vi "MDOAcquire Data from х502.vi"(8 "error in (no error)":errorcluster, 10 "Coeff":T2={"Coeff_U"=300.0, "Offset_U"=0.0, "Coeff_I"=23.5, "Offset_I"=0.15}, 11 "Hardware Configuration":T1 {"SyncMode" items=["INTERNAL"=0, "EXTERNAL_MASTER"=1, "DI_SYN1_RISE"=2, "DI_SYN1_FALL"=3, "DI_SYN2_RISE"=6, "DI_SYN2_FALL"=7]}) -> (0 "error out":errorcluster, 2 "Ток":dbl[](graph), 3 "Напряжение":dbl[](graph))   [LabVIEW 2012]
uses:
  controls/Coeff.ctl
  controls/MDOHW Configuration.ctl
  <vilib>/Analysis/3filter.llb/Filter Passband Type.ctl
  <vilib>/Analysis/3filter.llb/Butterworth Filter (DBL).vi
  <vilib>/Analysis/NI_AALBase.lvlib
panel:
  out "Gauge":dbl(knob) scale=0.0..10.0
  in  "stop":bool
  out "din_data_size":u32
  out "DIN":u32[](array[numeric]) format="%b"
  in  "IP Addr":string="192.168.0.1"
  out "MCU ver":string
  in  "Отображать за время":dbl=100.0 min=10.0 step=1.0
  out "Установленная частота синхронного ввода DIN":dbl=2.0 min=2.0 max=2000000.0 format="%#_8f"
  in  "Частота синхронного ввода DIN":dbl=20000.0 min=1.0 max=2000000.0 format="%#_8f"
  out "FPGA Ver":string
  out "Установленная частота на канал":dbl=2.0 min=2.0 max=2000000.0 format="%#_8f"
  out "Установленная частота сбора":dbl=2.0 min=2.0 max=2000000.0 format="%#_8f"
  in  "Частота сбора на канал":dbl=50000.0 min=2.0 max=2000000.0 format="%#_8f"
  in  "Частота сбора (Гц)":dbl=100000.0 min=2.0 max=2000000.0 format="%#_8f"
  out "PldaVer":u8
  out "Serial":string
  out "Name":string
  # "Ожидание триггера"
  # "Информация о плате"
  # "Настройки модуля"
  # "Устанавливаемое"
  # "Установленное"
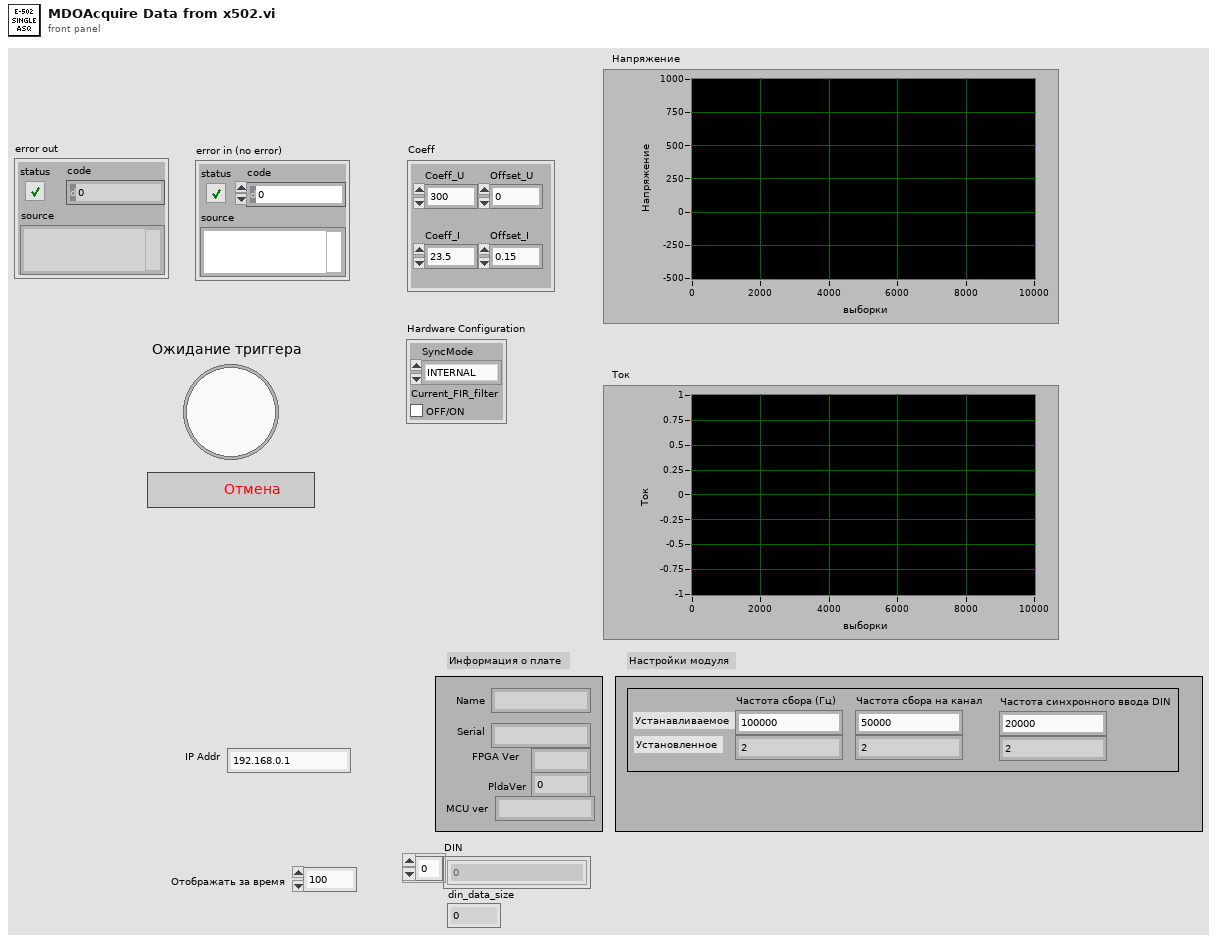
[diagram p1: front panel]
types:
  T1 = typedef "MDOHW Configuration.ctl" = cluster{"SyncMode":u32, "Current_FIR_filter":bool}
  T2 = typedef "Coeff.ctl" = cluster{"Coeff_U":dbl, "Offset_U":dbl, "Coeff_I":dbl, "Offset_I":dbl}
  T3 = cluster{"PhyCh":u32, "Avg":u32, "Mode":u32, "Range":u32}[]
  T4 = typedef "NI_AALBase.lvlib/Filter Passband Type.ctl" = enum32{"Lowpass", "Highpass", "Bandpass", "Bandstop"}
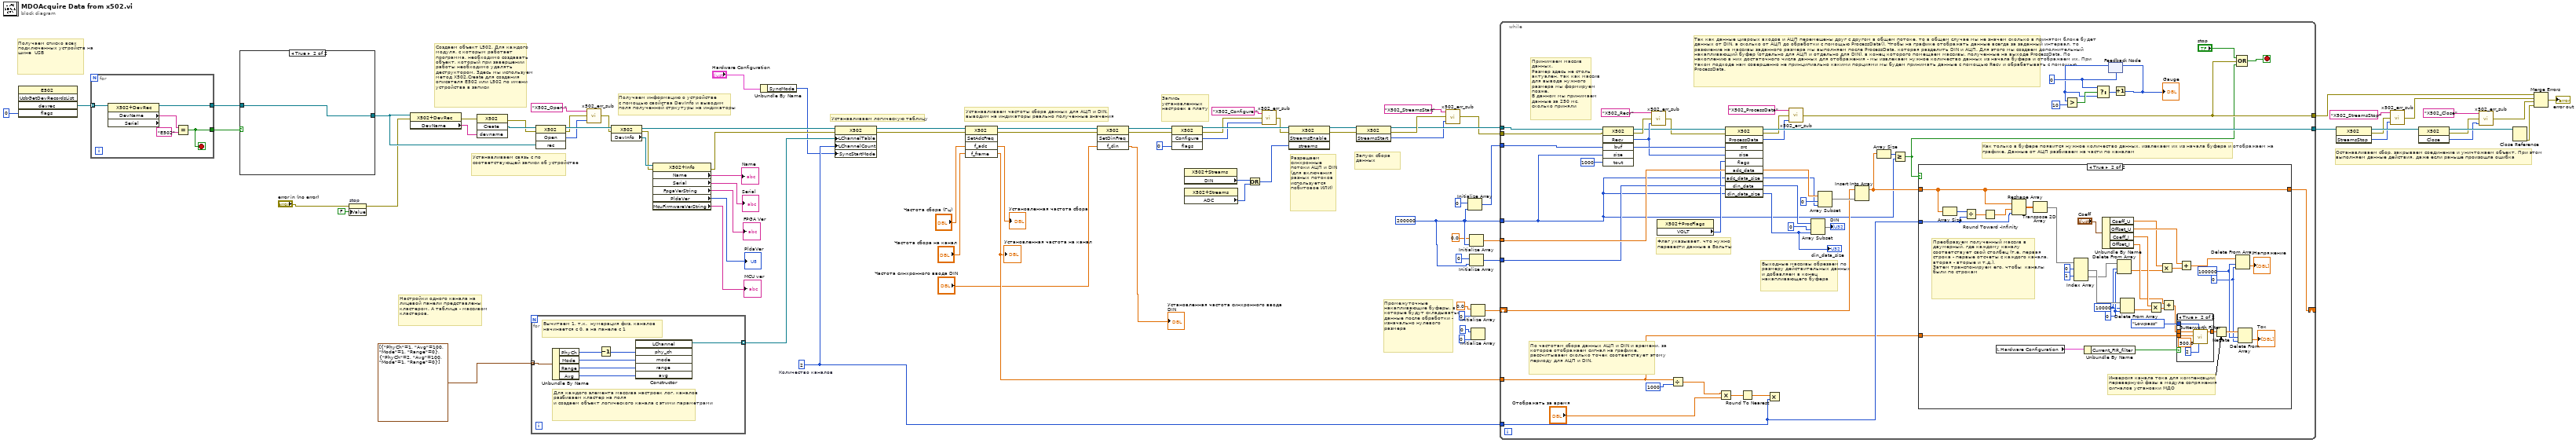
[diagram p0: block diagram]
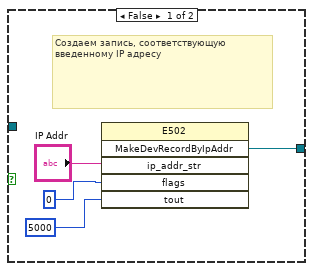
[diagram p4: hidden frame]
diagram:
  w85 = u32 2  # Количество каналов
  w81 = u32 200000 ("element")
  # "Промежуточные накапливающие буферы, в которые будут складываться данные после обработки - изначально нулевого размера"
  # "Получаем списко всех подключенных устройств на шине  USB"
  # "Останавливаем сбор, закрываем соединение и уничтожаем объект. При этом выполняем данные действия, даже если раньше произошла ошибка"
  # "Запуск сбора данных"
  # "Разрешаем синхронные потоки АЦП и DIN (для включения разных потоков используется побитовое ИЛИ)"
  # "Запись установленных настроек в плату"
  # "Устанавливаем частоты сбора данных для АЦП и DIN,\nвыводим на индикаторы реально полученные значения"
  # "Устанавливаем логическую таблицу"
  # "Настройки одного канала на лицевой панели представлены кластером. А таблица - массивом кластеров."
  # "Создаем объект L502. Для каждого модуля, с которым работает программа, необходимо создавать объект, который при завершении работы необходимо удалять деструктором. Здесь мы используем метод X502.Create для создания описателя E502 или L502 по имени устройства в записи"
  # "Получаем информацию о устройстве \nс помощью свойства DevInfo и выводим\nполя полученной стркутуры на индикаторы"
  # "Устанавливаем связь с по соответствующей записи об устройстве"
  n1 = invoke class="E502" method="UsbGetDevRecordsList"("flags"=0) -> ("devrec"=w15:refnum<k24>[])  [unwired: 4 in, 4 out]
  n2 = for {
    tunnel: w15 -> [w90] mode=indexing
    tunnel: [w89] -> w13
    tunnel: [w86] -> w14
    stop <- w86 stop-if-true
    n3 = property class="X502+DevRec" props=["DevName", "Serial"](reference=w90) -> (reference out=w89:refnum<k24>, "DevName"=w88:string)  [unwired: 1 in, 2 out]
    n4 = Equal?(x=w88, y="E502") -> (x = y?=w86:bool)
  }
  n5 = case shown="True" w14 {
    tunnel: [w91 w95] -> w22
    tunnel: w13 -> [_ w95]
    frame False {
      # "Создаем запись, соответствующую введенному IP адресу"
      n6 = invoke class="E502" method="MakeDevRecordByIpAddr"("ip_addr_str"="IP Addr", "flags"=0, "tout"=5000) -> ("MakeDevRecordByIpAddr"=w91:refnum<k24>)  [unwired: 3 in, 5 out]
    }
    frame True {
    }
  }
  n7 = property on="stop" class="Bool (strict)"(error in="error in (no error)", "Value"=FALSE ("Visible")) -> (error out=w10:errorcluster)  [unwired: 1 in, 1 out]
  n8 = property class="X502+DevRec"(reference=w22, error in=w10) -> (error out=w17:errorcluster, "DevName"=w53:string)  [unwired: 1 out]
  n9 = invoke class="X502" method="Create"(error in=w17, "devname"=w53) -> (error out=w52:errorcluster, "Create"=w54:refnum<k24>)  [unwired: 2 in, 2 out]
  n10 = for {
    tunnel: T3 [{"PhyCh"=1, "Avg"=100, "Mode"=1, "Range"=0}, {"PhyCh"=2, "Avg"=100, "Mode"=1, "Range"=0}] ("Логические каналы") -> [w102] mode=indexing
    tunnel: [w96] -> w77 mode=indexing
    # "Вычитаем 1, т.к.  нумерация физ. каналов начинается с 0, а на панеле с 1"
    # "Для каждого элемента массива настроек лог. каналов разбиваем кластер на поля\nи создаем объект логического канала с этими параметрами"
    n11 = Unbundle By Name(w102) -> ("PhyCh"=w101:u32, "Mode"=w99:u32, "Range"=w98:u32, "Avg"=w97:u32)
    n12 = Decrement(x=w101) -> (x-1=w100:u32)
    n13 = constructor class="X502+LChannel"("phy_ch"=w100, "mode"=w99, "range"=w98, "avg"=w97) -> (reference out=w96:refnum<k24>)  [unwired: 3 in, 6 out]
  }
  n14 = invoke class="X502" method="Open"(reference=w54, error in=w52, "rec"=w22) -> (reference out=w57:refnum<k24>, error out=w50:errorcluster, "Open"=w51:i32)  [unwired: 1 in, 1 out]
  n15 = call "x502_err_sub.vi"("Error code"=w51, "error in (no error)"=w50, "Error descr"="X502_Open ") -> ("error out"=w48:errorcluster)
  n16 = property class="X502"(reference=w57, error in=w48) -> (reference out=w58:refnum<k24>, error out=w46:errorcluster, "DevInfo"=w47:refnum<k24>)
  n17 = property class="X502+Info"(reference=w47, error in=w46) -> (error out=w23:errorcluster, "Name"=→"Name":string, "Serial"=→"Serial":string, "FpgaVerString"=→"FPGA Ver":string, "PldaVer"=→"PldaVer":u8, "McuFirmwareVerString"=→"MCU ver":string)  [unwired: 1 out]
  n18 = Unbundle By Name("Hardware Configuration") -> ("SyncMode"=w1:u32)
  n19 = property class="X502"(reference=w58, error in=w23, "LChannelTable"=w77, "LChannelCount"=w85, "SyncStartMode"=w1) -> (reference out=w59:refnum<k24>, error out=w60:errorcluster)
  n20 = invoke class="X502" method="SetAdcFreq"(reference=w59, error in=w60, "f_adc"="Частота сбора (Гц)", "f_frame"="Частота сбора на канал") -> (reference out=w64:refnum<k24>, error out=w65:errorcluster, "f_adc"=→"Установленная частота сбора":dbl, "f_frame"=w78:dbl)  [unwired: 1 in, 1 out]
  "Установленная частота на канал" <- w78
  n21 = invoke class="X502" method="SetDinFreq"(reference=w64, error in=w65, "f_din"="Частота синхронного ввода DIN") -> (reference out=w69:refnum<k24>, error out=w70:errorcluster, "f_din"=→"Установленная частота синхронного ввода DIN":dbl)  [unwired: 1 in, 1 out]
  n22 = invoke class="X502" method="Configure"(reference=w69, error in=w70, "flags"=0) -> (reference out=w71:refnum<k24>, error out=w40:errorcluster, "Configure"=w38:i32)  [unwired: 1 in, 1 out]
  n23 = property class="X502+Streams"() -> ("DIN"=w32:u32)  [unwired: 2 in, 2 out]
  n24 = property class="X502+Streams"() -> ("ADC"=w68:u32)  [unwired: 2 in, 2 out]
  n25 = Or(x=w32, y=w68) -> (x .or. y?=w31:u32)
  n26 = call "x502_err_sub.vi"("Error code"=w38, "error in (no error)"=w40, "Error descr"="X502_Configure ") -> ("error out"=w39:errorcluster)
  n27 = invoke class="X502" method="StreamsEnable"(reference=w71, error in=w39, "streams"=w31) -> (reference out=w72:refnum<k24>, error out=w73:errorcluster)  [unwired: 1 in, 2 out]
  n28 = invoke class="X502" method="StreamsStart"(reference=w72, error in=w73) -> (reference out=w34:refnum<k24>, error out=w36:errorcluster, "StreamsStart"=w8:i32)  [unwired: 1 in]
  n29 = call "x502_err_sub.vi"("Error code"=w8, "error in (no error)"=w36, "Error descr"="X502_StreamsStart") -> ("error out"=w33:errorcluster)
  n30 = Initialize Array(u32 0 ("element"), w81) -> (w82:u32[])
  n31 = Initialize Array(0.0 ("element"), w81) -> (w84:dbl[])
  n32 = Initialize Array(u32 0 ("element"), w81) -> (w83:u32[])
  n33 = Initialize Array(0.0 ("element"), u32 0 ("element")) -> (w3:dbl[])
  n34 = Initialize Array(u32 0 ("element"), u32 0 ("element")) -> ()  [unwired: 1 out]
  n35 = while {
    tunnel: w85 -> [w149]
    tunnel: w84 -> [w148]
    tunnel: w83 -> [w147]
    tunnel: w82 -> [w146]
    tunnel: w81 -> [w104]
    tunnel: w78 -> [w113]
    tunnel: w34 -> [w145]
    tunnel: w33 -> [w144]
    tunnel: [w143] -> w30
    tunnel: [w121] -> w18
    shift-right: [w107] -> _
    shift-left: w3 -> [w108]
    stop <- w120 stop-if-true
    w116 = 0
    # "Так как данные цивроых входов и АЦП перемешены друг с другом в общем потоке, то в общем случае мы не значем сколько в принятом блоке будет данных от DIN, а сколько от АЦП до обработки с помощью ProcessData(). Чтобы на графике отображать данные всегда за заданный интервал, то разюиение на массивы заданного размера мы выполняем после ProcessData, которая разделить DIN и АЦП. Для этого мы создаем дополнительный накапливающий буфер (отдельно для АЦП и отдельно для DIN), в конец которого помещаем массивы, полученные на выходе ProcessData. По накоплению в них достаточного числа данных для отображения - мы извлекаем нужное количество данных из начала буфера и отображаем их. При таком подходе нам совершенно не принципиально какими порциями мы будем принимать данные с помощью Recv и обрабатывать с помощью ProcessData."
    # "Как только в буфере появится нужное количество данных, извлекаем их из начала буфера и отображаем на графике. Данные от АЦП разбиваем на части по каналам"
    # "По частотам сбора данных АЦП и DIN и времени, за которое отображаем сигнал на графике, рассчитываем сколько точек соответствует этому периоду для АЦП и DIN."
    # "Выходные массивы обрезаем по размеру действительных данных и добавляем в конец накапливающего буфера"
    # "Флаг указывает, что нужно перевести данные в Вольты"
    # "Принимаем массив данных.\nРазмер здесь не столь актуален, так как массив для вывода нужного размера мы формируем позже.\nВ данном мы принимаем данные за 250 мс, сколько приняли"
    n36 = invoke class="X502" method="Recv"(reference=w145, error in=w144, "buf"=w146, "size"=w104, "tout"=u32 1000 ("element")) -> (reference out=w124:refnum<k24>, error out=w130:errorcluster, "Recv"=w129:i32, "buf"=w142:u32[])  [unwired: 1 in, 2 out]
    n37 = call "x502_err_sub.vi"("Error code"=w129, "error in (no error)"=w130, "Error descr"="X502_Recv") -> ("error out"=w123:errorcluster)
    n38 = property class="X502+ProcFlags"() -> ("VOLT"=w140:u32)  [unwired: 2 in, 2 out]
    n39 = Divide(x=w113, y=1000) -> (x/y=w135:dbl)
    n40 = Multiply(x=w135, y="Отображать за время") -> (x*y=w134:dbl)
    n41 = invoke class="X502" method="ProcessData"(reference=w124, error in=w123, "src"=w142, "size"=w129, "flags"=w140, "adc_data"=w148, "adc_data_size"=w104, "din_data"=w147, "din_data_size"=w104) -> (reference out=w143:refnum<k24>, error out=w127:errorcluster, "ProcessData"=w126:i32, "adc_data"=w112:dbl[], "adc_data_size"=w110:u32, "din_data"=w138:u32[], "din_data_size"=w137:u32)  [unwired: 1 in, 3 out]
    "din_data_size" <- w137
    n42 = Round To Nearest(number=w134) -> (nearest integer value=w133:dbl)
    n43 = Multiply(x=w133, y=w149) -> ()  [unwired: 1 out]
    n44 = call "x502_err_sub.vi"("Error code"=w126, "error in (no error)"=w127, "Error descr"="X502_ProcessData") -> ("error out"=w121:errorcluster)
    n45 = Array Subset(array=w138, index=u32 0 ("element"), length=w137) -> (→"DIN":u32[])
    n46 = Array Subset(array=w112, index=0, length=w110) -> (w109:dbl[])
    n47 = Insert Into Array(array=w108, new element=w109) -> (w106:dbl[])  [unwired: 1 in]
    n48 = Array Size(array=w106) -> (size(s)=w105:i32)
    n49 = Greater Or Equal?(x=w105, y=w104) -> (x >= y?=w103:bool)
    n50 = case shown="True" w103 {
      tunnel: w149 -> [_ w184]
      tunnel: w113 -> [_ w176]
      tunnel: w106 -> [w150 w153]
      tunnel: [w150 w153] -> w107
      frame False {
      }
      frame True {
        w155 = 0 ("index")
        w156 = 100000 ("length")
        w162 = 0 ("index")
        w161 = 10000 ("length")
        # "Инверсия канала тока для компенсации \nперевернуой фазы в модуле сопряжения \nсигналов установки МДО"
        # "Преобразуем полученный массив в двумерный, где каждому каналу соответствует свой столбец (т.е. первая строка - первые отсчеты с каждого канала, вторая - вторые и т.д.).\nЗатем транспонируем его, чтобы  каналы были по строкам"
        n51 = Array Size(array=w153) -> (size(s)=w154:i32)
        n52 = Divide(x=w154, y=w184) -> (x/y=w183:dbl)
        n53 = Round Toward -Infinity(1:w183) -> (0:w182:dbl)
        n54 = local read "Hardware Configuration"() -> (w152:T1)
        n55 = Reshape Array(w153, w182, w184) -> (w177:dbl[][])
        n56 = Transpose 2D Array(2D array=w177) -> (transposed array=w167:dbl[][])
        n57 = Index Array(array=w167, index (row) #1=0 ("index (row)"), index (row) #2=1 ("index (row)")) -> (element #1=w166:dbl[], element #2=w163:dbl[])  [unwired: 2 in]
        n58 = Unbundle By Name(w152) -> ("Current_FIR_filter"=w151:bool)
        n59 = Unbundle By Name("Coeff") -> ("Coeff_U"=w170:dbl, "Offset_U"=w171:dbl, "Coeff_I"=w169:dbl, "Offset_I"=w168:dbl)
        n60 = Delete From Array(array=w163, length=w161, index=w162) -> (deleted portion=w164:dbl[])  [unwired: 1 out]
        n61 = Delete From Array(array=w166, length=w161, index=w162) -> (deleted portion=w165:dbl[])  [unwired: 1 out]
        n62 = Multiply(x=w169, y=w165) -> (x*y=w179:dbl[])
        n63 = Multiply(x=w170, y=w164) -> (x*y=w178:dbl[])
        n64 = Add(x=w168, y=w179) -> (x+y=w174:dbl[])
        n65 = case shown="True" w151 {
          tunnel: w176 -> [_ w191]
          tunnel: Filter_Passband_Type."Lowpass" ("filter type") -> [_ w190]
          tunnel: w174 -> [w185 w188]
          tunnel: [w185 w186] -> w173
          frame False {
          }
          frame True {
            n66 = call-poly <vilib>:"Butterworth Filter.vi"("order"=2, "filter type"=w190, "low cutoff freq: fl"=500.0, "sampling freq: fs"=w191, "X"=w188) -> ("Filtered X"=w186:dbl[])  [unwired: 3 in, 1 out]
          }
        }
        n67 = Add(x=w171, y=w178) -> (x+y=w160:dbl[])
        n68 = Negate(x=w173) -> (-x=w158:dbl[])
        n69 = Delete From Array(array=w160, length=w156, index=w155) -> (deleted portion=→"Напряжение":dbl[])  [unwired: 1 out]
        n70 = Delete From Array(array=w158, length=w156, index=w155) -> (deleted portion=→"Ток":dbl[])  [unwired: 1 out]
      }
    }
    n71 = feedback #1(w116) -> (w115:i32)
    n72 = Greater?(x=w115, y=10) -> (0:w117:bool)
    n73 = Select(t=w116, s=w117, f=w115) -> (s? t:f=w114:i32)
    n74 = Increment(x=w114) -> (x+1=w119:i32)
    "Gauge" <- w119
    n75 = feedback-in #1(w119) -> ()
    n76 = Compound Arithmetic op=OR("stop", w121, w103) -> (w120:bool)
  }
  n77 = invoke class="X502" method="StreamsStop"(reference=w30) -> (reference out=w55:refnum<k24>, error out=w29:errorcluster, "StreamsStop"=w27:i32)  [unwired: 2 in]
  n78 = call "x502_err_sub.vi"("Error code"=w27, "error in (no error)"=w29, "Error descr"="X502_StreamsStop") -> ("error out"=w19:errorcluster)
  n79 = invoke class="X502" method="Close"(reference=w55) -> (reference out=w56:refnum<k24>, error out=w25:errorcluster, "Close"=w24:i32)  [unwired: 2 in]
  n80 = call "x502_err_sub.vi"("Error code"=w24, "error in (no error)"=w25, "Error descr"="X502_Close") -> ("error out"=w20:errorcluster)
  n81 = Close Reference(reference=w56) -> (error out=w21:errorcluster)  [unwired: 1 in]
  n82 = Merge Errors(w18, w19, w20, w21) -> (→"error out":errorcluster)
